vi "IQ_PID.vi"(0 "Data in":fxp<+/-,16,14>[](array[numeric])=[0.0, 0.0, 0.0, 0.0], 1 "Ki*Tau I":fxp<+/-,32,6>, 2 "Kp I":fxp<+/-,32,6>, 3 "Kd/Tau I":fxp<+/-,32,6>, 5 "Enable I":bool=TRUE, 7 "Enable Q":bool=TRUE, 9 "Reset":bool=TRUE, 11 "input valid":bool=TRUE, 12 "Ki*Tau Q":fxp<+/-,32,6>, 13 "Kp Q":fxp<+/-,32,6>, 14 "Kd/Tau Q":fxp<+/-,32,6>) -> (4 "data out":fxp<+/-,16,14>[](array[numeric]), 10 "output valid":bool)   [LabVIEW 2018]
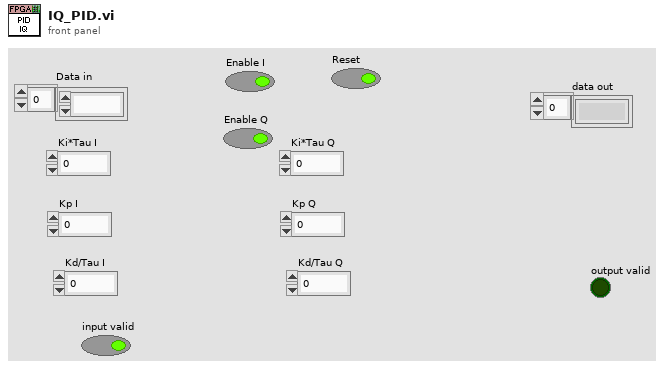
[diagram p1: front panel]
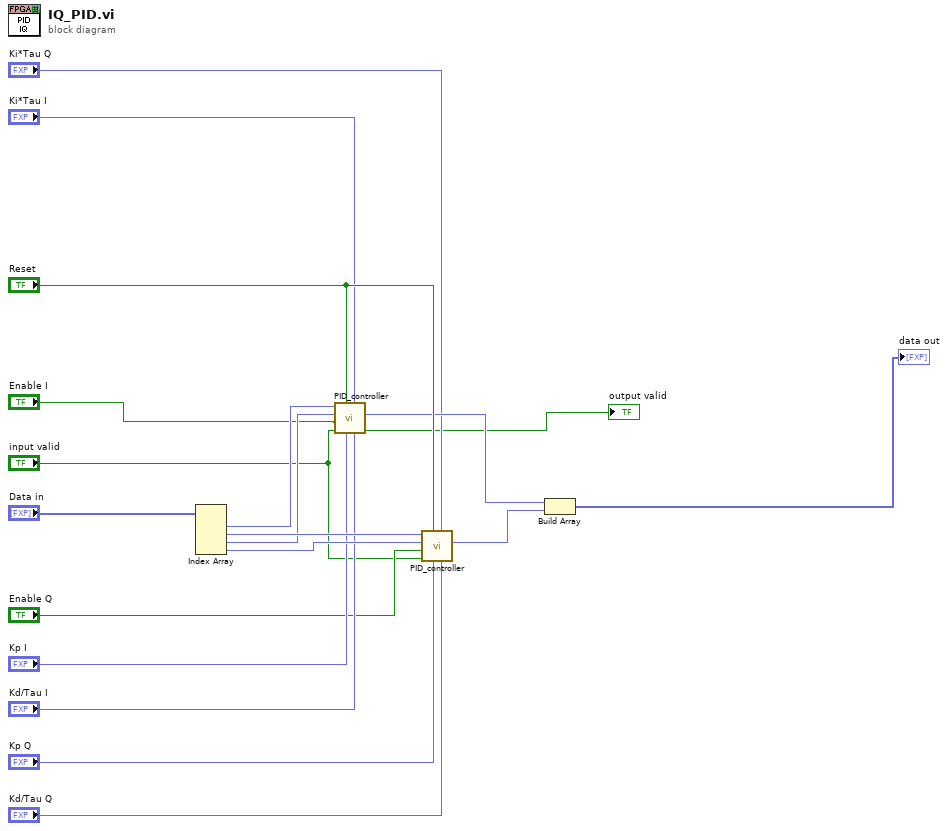
[diagram p0: block diagram]
diagram:
  n1 = Index Array(array="Data in") -> (element #1=w18:fxp<+/-,16,14>, element #2=w17:fxp<+/-,16,14>, element #3=w16:fxp<+/-,16,14>, element #4=w15:fxp<+/-,16,14>)  [unwired: 4 in]
  n2 = call "PID_controller.vi"("Kd/Tau"="Kd/Tau I", "Ki*Tau"="Ki*Tau I", "Kp"="Kp I", "Reset"="Reset", "input valid"="input valid", "Enabled"="Enable I", "Y in"=w16, "Ref in"=w18) -> ("output valid"=→"output valid":bool, "Y out"=w9:fxp<+/-,16,14>)  [unwired: 1 in, 1 out]
  n3 = call "PID_controller.vi"("Kd/Tau"="Kd/Tau Q", "Ki*Tau"="Ki*Tau Q", "Kp"="Kp Q", "Reset"="Reset", "input valid"="input valid", "Enabled"="Enable Q", "Y in"=w15, "Ref in"=w17) -> ("Y out"=w8:fxp<+/-,16,14>)  [unwired: 1 in, 2 out]
  n4 = Build Array(w9, w8) -> (→"data out":fxp<+/-,16,14>[])
